vi "main_set_simulation_file.vi"(10 "Simulation file":refnum<vi>, 11 "Running?":refnum<vi>) -> ()   [LabVIEW 2019]
uses:
  lib/libSimulationControl/libSimulationControl.lvlib
panel:
  # "*******************************************************************\nBiogas Plant Control\n\nAuthor: Paul Zügel\nGCSC-Frankfurt am Main 2020\n\n*******************************************************************"
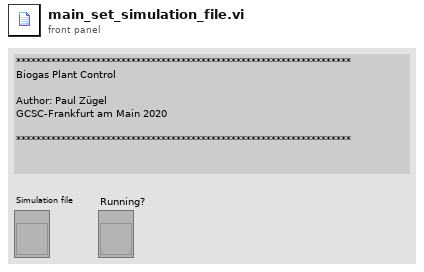
[diagram p1: front panel]
types:
  T1 = enum8{"Enabled", "Disabled", "Disabled and Grayed Out"}
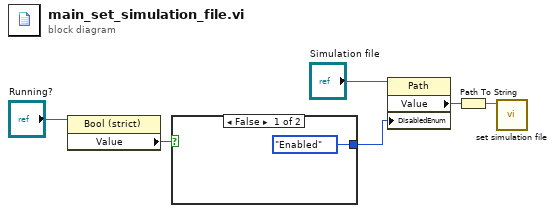
[diagram p0: block diagram]
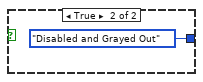
[diagram p2: hidden frame]
diagram:
  n1 = property class="Bool (strict)"(reference="Running?") -> ("Value"=w2:bool)  [unwired: 1 in, 2 out]
  n2 = case shown="False" w2 {
    tunnel: [T1."Enabled" ("Disabled") T1."Disabled and Grayed Out" ("Disabled")] -> w6
    frame False {
    }
    frame True {
    }
  }
  n3 = property class="Path"(reference="Simulation file", "DisabledEnum"=w6) -> ("Value"=w4:path)  [unwired: 1 in, 2 out]
  n4 = Path To String(path=w4) -> (string=w3:string)
  n5 = call "set simulation file.vi"("sim_file"=w3) -> ()  [unwired: 10 in, 1 out]
